vi "SOUR_POW_CORR_COLL_TABL_LOSS_STAT.vi"(0 "VISA IN":refnum<visa-resource-name>, 1 "Loss Table ON/OFF":bool, 5 "error in":errorcluster, 7 "Channel":i32) -> (14 "VISA Out":refnum<visa-resource-name>, 19 "error out":errorcluster)   [LabVIEW 2018, in "PNA-X.lvlib"]
doc: "SOURce<cnum>:POWer:CORRection:COLLect:TABLe:LOSS[:STATe] <ON | OFF> \n1844\n\n(Read-Write) Indicates whether or not to adjust the power readings using the values in the loss table \nduring a source power cal sweep. \nParameters \n<cnum> Any existing channel number. If unspecified, value is set to 1 \n<ON|OFF> ON (or 1) - turns use of the loss table ON. \nOFF (or 0) - turns use of the loss table OFF. \nExamples SOUR:POW:CORR:COLL:TABL:LOSS ON \nsource1:power2:correction:collect:table:loss:state off \nQuery Syntax SOURce:POWer:CORRection:COLLect:TABLe:LOSS[:STATe]? \nReturn Type Boolean (1 = ON, 0 = OFF) \nDefault OFF (0)"
uses:
  PNA-X.lvlib
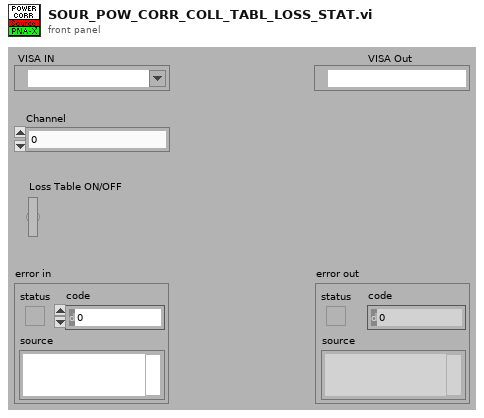
[diagram p1: front panel]
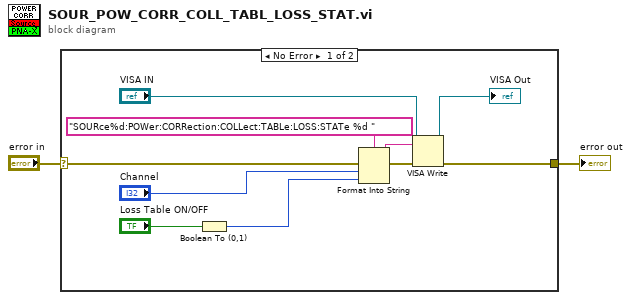
[diagram p0: block diagram]
diagram:
  n1 = case shown="No Error" "error in" {
    selector: "error in" -> [w12 w13]
    tunnel: [w7 w13] -> w1
    frame No Error {
      n2 = Boolean To (0,1)(Boolean="Loss Table ON/OFF") -> (0, 1=w3:i16)
      n3 = Format Into String(format string="SOURce%d:POWer:CORRection:COLLect:TABLe:LOSS:STATe %d " ("Cmdline"), error in=w12, "Channel", w3) -> (resulting string=w10:string, error out=w11:errorcluster)  [unwired: 1 in]
      n4 = VISA Write(VISA resource name="VISA IN", write buffer=w10, error in (no error)=w11) -> (VISA resource name out=→"VISA Out":refnum<visa-resource-name>, error out=w7:errorcluster)  [unwired: 1 out]
    }
    frame Error {
    }
  }
  "error out" <- w1
